vi "g2Cal 80 MHz with random input.vi"() -> ()   [LabVIEW 2015]
uses:
  <vilib>/Platform/TimedLoop/XDataNode/timing_clust.ctl
  <vilib>/Platform/TimedLoop/XDataNode/nitl_modes.ctl
  <vilib>/Platform/TimedLoop/XDataNode/wakeup.ctl
  <vilib>/rvi/Emulation/niFpgaGetClockAttributes.vi
  <vilib>/rvi/Emulation/niFpgaSctlEmulationGetInTimedLoop.vi
  <vilib>/rvi/Emulation/niFpgaEmulationReportErrorSimple.vi
  <vilib>/rvi/DataTransferAndStorage/Container/Common/niFpgaContainerGetUniqueNameForEmu.vi
  <vilib>/rvi/DataTransferAndStorage/Container/Common/niFpgaContainerSetEmuInfo.vi
  <vilib>/rvi/eio/common/nirviEmuReportErrorAndStop.vi
  <vilib>/rvi/Emulation/niFpgaCriticalErrorInLSC.vi
  Tick Count (U64) Global.vi
  <vilib>/rvi/DataTransferAndStorage/Container/Common/niFpgaContainerExecOnDevCompGetState.vi
  <vilib>/rvi/Emulation/niFpgaEmulationIsFPGAContextNoSignature.vi
  <vilib>/rvi/errors/niFpgaSetErrorForExecOnDevCompSimple.vi
  <vilib>/rvi/FIFO/Fifo_Resource/nirvififoEmulationSetSize.vi
  <vilib>/rvi/FIFO/Fifo_Resource/nirviFifoEmulationQueueMgr.vi
  <instcachedir>/0/nirviFifoEmulationQueueMgr_E5CAEC123FF24DC58D834DCA3CDAA9B5.lvgen/nirviFifoEmulationQueueMgr_E5CAEC123FF24DC58D834DCA3CDAA9B5_000.vi
  <vilib>/rvi/FIFO/Fifo_Resource/nirvififoEmulationDetermineInputValidOut.vi
  <vilib>/rvi/FIFO/Fifo_Resource/nirvififoEmulationCreateLock.vi
  <vilib>/rvi/Emulation/niFpgaProcessEmulError.vi
  <vilib>/rvi/FIFO/Fifo_Resource/nirvififoEmulationObtainLock.vi
  <vilib>/rvi/FIFO/Fifo_Resource/nirvififoEmulationReleaseLock.vi
  <vilib>/rvi/occurrence/nirviWaitOnOccurrenceBase.vi
  <vilib>/rvi/errors/nirviReportUnexpectedCaseInternalError.vi
  <vilib>/rvi/errors/nirviReportUnexpectedCaseInternalError (U32).vi
  <vilib>/Utility/error.llb/Clear Errors.vi
  <vilib>/rvi/interface/RandomDataEmulation/niFpgaRandomDataHandleErrors.vi
  <vilib>/rvi/eio/common/nirviEmuTemplateMethod_errors.vi
  <vilib>/Platform/TimedLoop/XDataNode/XDataNode.xnode
  <vilib>/rvi/LocalResourceManager/LocalResourceManager.xnode
  <vilib>/rvi/FXPMathLib/FxpMul/XNode/nifxpmath_Multiplier.xnode
  <vilib>/rvi/FXPMathLib/FxpSub/XNode/nifxpmath_Sub.xnode
  <vilib>/rvi/DataTransferAndStorage/Container/XNode/niFpgaContainer.xnode
  <vilib>/rvi/FIFO/Fifo_Resource/niFpgaFifoEmulationRefIn.vi
  <vilib>/eio/EIONode/EIONode.xnode
  <vilib>/rvi/interface/RandomDataEmulation/nirviRandomDataFpgaReadWriteTemplate.vi
  <vilib>/Platform/TimedLoop/XDataNode/XDNodeRunTimeDep.lvlib
  <vilib>/rvi/FXPMathLib/sim/FxpSim.dll
panel:
  in  "Random":bool
  in  "Frequency (MHz)":fxp<+,32,4>=0.006250001490116119
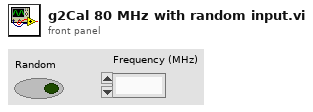
[diagram p1: front panel]
types:
  T1 = typedef "XDNodeRunTimeDep.lvlib/timing_clust.ctl" = cluster{"Expected End [f-1]":u64, "Actual End [f-1]":u64, "Finished Late? [f-1]":bool, "Expected End [i-1]":u64, "Actual End [i-1]":u64, "Finished Late? [i-1]":bool, "Expected Start [i]":u64, "Actual Start [i]":u64, "Expected Start [f]":u64, "Actual Start [f]":u64, "Source Name":string, "Structure Name":string, "Period":i64, "Deadline":i64, "Offset":i64, "Start":i64, "Priority":i32, "Timeout":i32, "Mode":T2, "Wakeup Reason":T3, "Error":errorcluster, "Source Type":string, "Secondary Source Type":string, "Global End Time":u64, "Global Start Time":u64, "Frame Duration":u64, "Iteration Duration":u64, "Assigned CPU":i32, "I/O Scan Engine Mode":u32}
  T2 = typedef "XDNodeRunTimeDep.lvlib/nitl_modes.ctl" = enum32{"No Change", "Process missed periods, maintain original phase", "Discard missed periods, maintain original phase", "Process missed periods, ignore original phase", "Discard missed periods, ignore original phase"}
  T3 = typedef "XDNodeRunTimeDep.lvlib/wakeup.ctl" = enum32{"Normal", "Aborted", "Asynchronous wakeup", "Timing source error", "Timed loop error", "Timeout"}
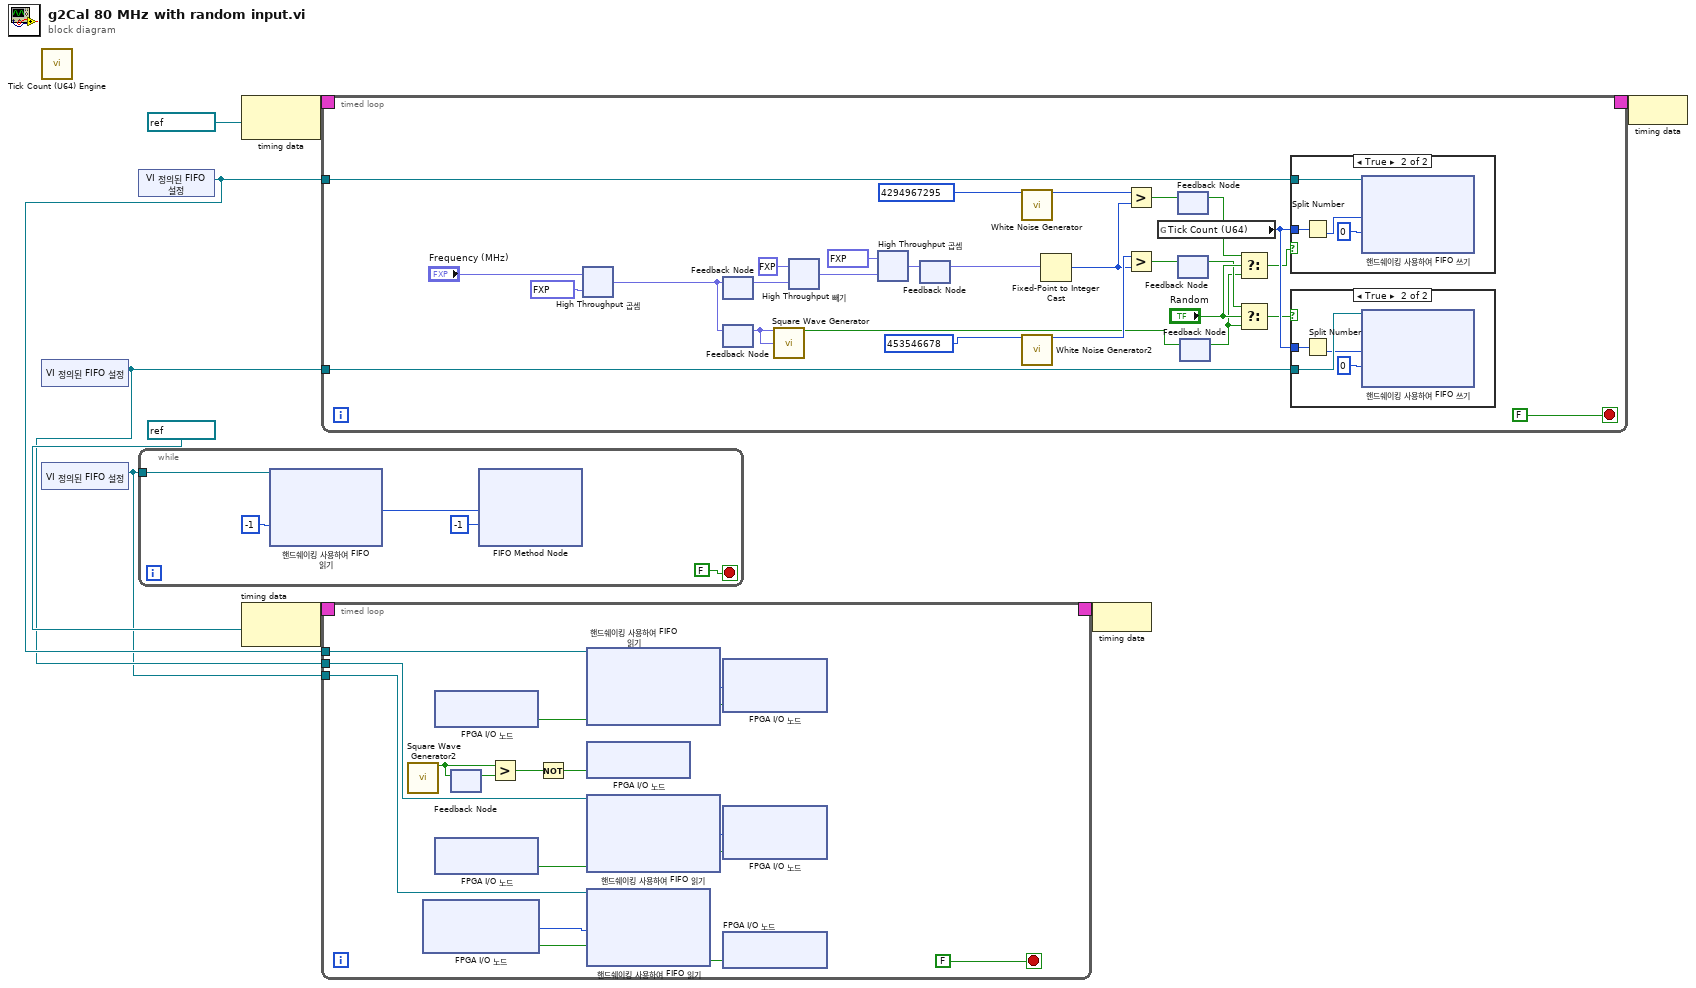
[diagram p0: block diagram]
diagram:
  n1 = call "Tick Count (U64) Engine.vi"() -> ()  [unwired: 1 in]
  n2 = xnode "VI 정의된 FIFO 설정"() -> ("FIFO Out"=w3:refnum<k21>)
  n3 = xnode "VI 정의된 FIFO 설정"() -> ("FIFO Out"=w1:refnum<k21>)
  n4 = xnode "VI 정의된 FIFO 설정"() -> ("FIFO Out"=w4:refnum<k21>)
  n5 = while {
    tunnel: w1 -> [w14]
    stop <- FALSE stop-if-true
    n6 = xnode ("핸드쉐이킹 사용하여 FIFO 읽기")("Timeout"=-1 ("타임아웃"), "FIFO In"=w14) -> ("Element"=w12:u32)  [unwired: 2 out]
    n7 = xnode ("FIFO Method Node")("Element"=w12, "Timeout"=-1 ("타임아웃")) -> ()  [unwired: 1 in, 2 out]
  }
  n8 = node-c288(refnum<k21> "80MHz" ("소스 이름")) -> (w6:T1)
  n9 = node-c288(refnum<k21> "80MHz" ("소스 이름")) -> (w9:T1)
  n10 = timed-loop {
    timing: w6 -> [_]
    timing-out: [_] -> w5
    tunnel: w4 -> [w42]
    tunnel: w3 -> [w41]
    stop <- FALSE stop-if-true
    n11 = xnode ("High Throughput 곱셈")("x"="Frequency (MHz)", "y"=fxp<+,32,0> 0.012499999953433871) -> ("x*y"=w15:fxp<+,32,0>)
    n12 = feedback #1() -> (w16:fxp<+,32,0>)  [unwired: 1 in]
    n13 = feedback-in #1(w15) -> ()
    n14 = feedback-in #2(w15) -> ()
    n15 = feedback #2() -> (w25:fxp<+,32,0>)  [unwired: 1 in]
    n16 = call "Square Wave Generator"("frequency (periods/tick)"=w25, "duty cycle (periods)"=w25) -> ("square wave out"=w22:bool)  [unwired: 13 in]
    n17 = xnode "High Throughput 빼기"("x"=fxp<+,32,0> 0.9999999997671694, "y"=w16) -> ("x-y"=w28:fxp<+,32,0>)
    n18 = xnode ("High Throughput 곱셈")("x"=fxp<+,16,16> 32786.0, "y"=w28) -> ("x*y"=w24:fxp<+/-,16,16>)
    n19 = feedback #3() -> (w23:fxp<+/-,16,16>)  [unwired: 1 in]
    n20 = feedback-in #3(w24) -> ()
    n21 = call "White Noise Generator"("seed"=u32 4294967295) -> ("white noise out"=w37:i16)  [unwired: 14 in]
    n22 = call "White Noise Generator2"("seed"=u32 453546678) -> ("white noise out"=w33:i16)  [unwired: 14 in]
    n23 = Fixed-Point to Integer Cast(1:w23) -> (0:w26:i16)
    n24 = Greater?(x=w37, y=w26) -> (0:w20:bool)
    n25 = Greater?(x=w33, y=w26) -> (0:w21:bool)
    n26 = global read "Tick Count (U64) Global.vi" "Tick Count (U64)"() -> (w38:u64)
    n27 = feedback #4() -> (w19:bool)  [unwired: 1 in]
    n28 = feedback-in #4(w20) -> ()
    n29 = feedback #5() -> (w18:bool)  [unwired: 1 in]
    n30 = feedback-in #5(w21) -> ()
    n31 = feedback #6() -> (w17:bool)  [unwired: 1 in]
    n32 = feedback-in #6(w22) -> ()
    n33 = Select(t=w19, s="Random", f=w17) -> (s? t:f=w31:bool)
    n34 = Select(t=w18, s="Random", f=w17) -> (s? t:f=w30:bool)
    n35 = case shown="True" w31 {
      tunnel: w42 -> [_ w50]
      tunnel: w38 -> [_ w49]
      frame False {
      }
      frame True {
        n36 = Split Number(x=w49) -> (lo(x)=w47:u32)  [unwired: 1 out]
        n37 = xnode ("핸드쉐이킹 사용하여 FIFO 쓰기")("Element"=w47, "Timeout"=0 ("타임아웃"), "FIFO In"=w50) -> ()  [unwired: 2 out]
      }
    }
    n38 = case shown="True" w30 {
      tunnel: w41 -> [_ w46]
      tunnel: w38 -> [_ w43]
      frame False {
      }
      frame True {
        n39 = Split Number(x=w43) -> (lo(x)=w44:u32)  [unwired: 1 out]
        n40 = xnode ("핸드쉐이킹 사용하여 FIFO 쓰기")("Element"=w44, "Timeout"=0 ("타임아웃"), "FIFO In"=w46) -> ()  [unwired: 2 out]
      }
    }
  }
  n41 = timed-loop {
    timing: w9 -> [_]
    timing-out: [_] -> w8
    tunnel: w4 -> [w69]
    tunnel: w3 -> [w68]
    tunnel: w1 -> [w56]
    stop <- FALSE stop-if-true
    n42 = call "Square Wave Generator2"() -> ("square wave out"=w66:bool)  [unwired: 15 in]
    n43 = xnode "FPGA I/O 노드"() -> ("g2Cal\\g2Dat"=w55:u32, "g2Cal\\g2V"=w54:bool)  [unwired: 2 in, 2 out]
    n44 = xnode "FPGA I/O 노드"() -> ("g2Cal\\a1R"=w63:bool)  [unwired: 1 in, 1 out]
    n45 = xnode "FPGA I/O 노드"() -> ("g2Cal\\a2R"=w57:bool)  [unwired: 1 in, 1 out]
    n46 = feedback #7() -> (w67:bool)  [unwired: 1 in]
    n47 = feedback-in #7(w66) -> ()
    n48 = Greater?(x=w66, y=w67) -> (0:w65:bool)
    n49 = Not(x=w65) -> (.not. x?=w60:bool)
    n50 = xnode ("핸드쉐이킹 사용하여 FIFO 읽기")("Ready for Output"=w63, "FIFO In"=w69) -> ("Element"=w62:u32, "Output Valid"=w61:bool)  [unwired: 1 out]
    n51 = xnode "FPGA I/O 노드"("g2Cal\\RST"=w60) -> ()  [unwired: 1 in, 1 out]
    n52 = xnode ("핸드쉐이킹 사용하여 FIFO 읽기")("Ready for Output"=w57, "FIFO In"=w68) -> ("Element"=w59:u32, "Output Valid"=w58:bool)  [unwired: 1 out]
    n53 = xnode ("핸드쉐이킹 사용하여 FIFO 읽기")("Element"=w55, "Input Valid"=w54, "FIFO In"=w56) -> ("Ready for Input"=w53:bool)  [unwired: 1 out]
    n54 = xnode "FPGA I/O 노드"("g2Cal\\a1"=w62, "g2Cal\\a1V"=w61) -> ()  [unwired: 2 in, 2 out]
    n55 = xnode "FPGA I/O 노드"("g2Cal\\a2"=w59, "g2Cal\\a2V"=w58) -> ()  [unwired: 2 in, 2 out]
    n56 = xnode "FPGA I/O 노드"("g2Cal\\g2R"=w53) -> ()  [unwired: 1 in, 1 out]
  }
  n57 = node-c288(w8) -> ()
  n58 = node-c288(w5) -> ()
